vi "PanelB.vi"(0 "Numeric Control":dbl=54.6, 5 "Boolean Control":bool=TRUE, 7 "String Control":string="ABCD34EFGH") -> (4 "Numeric Indicator":dbl=54.6, 6 "Boolean Indicator":bool=TRUE, 8 "String Indicator":string="ABCD34EFGH")   [LabVIEW 2020, in "GetControlDetailsTests.lvlib"]
doc: "This VI has three types of controls and indicators"
uses:
  GetControlDetailsTests.lvlib
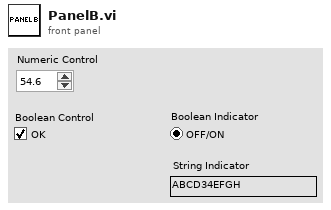
[diagram p1: front panel]
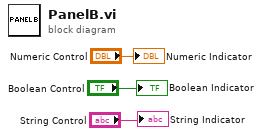
[diagram p0: block diagram]
diagram:
  "Numeric Indicator" <- "Numeric Control"
  "Boolean Indicator" <- "Boolean Control"
  "String Indicator" <- "String Control"
